vi "Send Configure Alarms.vi"(6 "Boolean Alarm Controls":T1, 7 "Message Priority (Normal)":T3=enum."Normal", 8 "error in (no error)":errorcluster, 9 "Alarm Limits":T2 {"Deadband (0.0000)" min=0.0 max=9999.9 step=0.0001 format="%.4f"; "Low Value (0.0000)" min=-9999.9 max=9999.9 step=0.0001 format="%.4f"; "High Value (0.0000)" min=-9999.9 max=9999.9 step=0.0001 format="%.4f"}, 10 "Input (0)":i32 min=0 max=7 step=1, 11 "Message Enqueuer":refnum<class "Message Enqueuer.lvclass">) -> (0 "error out":errorcluster, 3 "Message Enqueuer out":refnum<class "Message Enqueuer.lvclass">)   [LabVIEW 2016, in "LS218.lvlib" / "Configure Alarms Msg.lvclass"]
doc: "Sends the <B>LS218.lvlib:Configure Alarms Msg.lvclass</B> message.\n\n<B>LS218.lvlib:LS218.lvclass:Configure Alarms.vi</B> Description:\n\nThis VI configures all alarm functions for the selected input. Alarm functions include source, on/off, high value, low value, deadband, and latching parameters. This VI also enables/disables the system beeper, this control applies to all inputs."
uses:
  Configure Alarms Msg.lvclass
  <vilib>/ActorFramework/Message Enqueuer/Message Enqueuer.lvclass
  <vilib>/ActorFramework/Message Enqueuer/Message Priority.ctl
  C:/Program Files (x86)/National Instruments/LabVIEW 2016/vi.lib/ActorFramework/Message/Message.lvclass
  Configure Alarms Msg.lvclass/Configure Alarms Msg.ctl
  <vilib>/ActorFramework/Message Enqueuer/Message Enqueuer.lvclass/Message Enqueuer.ctl
  <vilib>/ActorFramework/Message Priority Queue/Priority Enqueue.vi
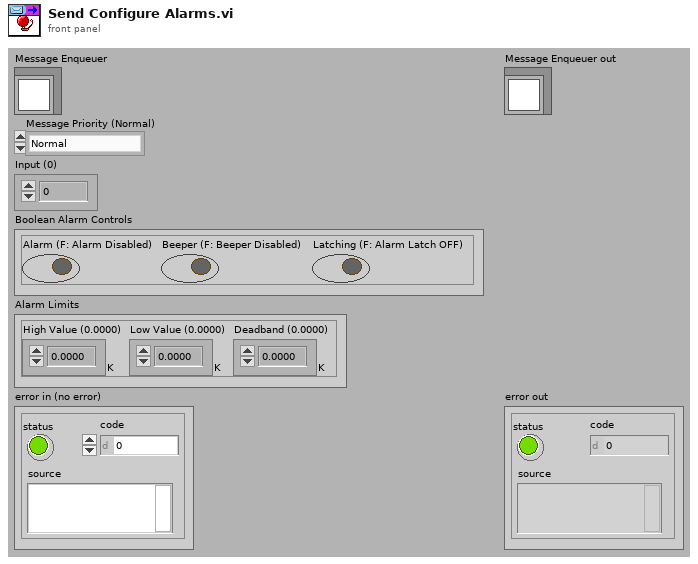
[diagram p1: front panel]
types:
  T1 = cluster{"Alarm (F: Alarm Disabled)":bool, "Beeper (F: Beeper Disabled)":bool, "Latching (F: Alarm Latch OFF)":bool}
  T2 = cluster{"High Value (0.0000)":dbl[unit], "Low Value (0.0000)":dbl[unit], "Deadband (0.0000)":dbl[unit]}
  T3 = typedef "Actor Framework.lvlib/Message Enqueuer.lvclass/Message Priority.ctl" = enum16{"Low", "Normal", "High"}
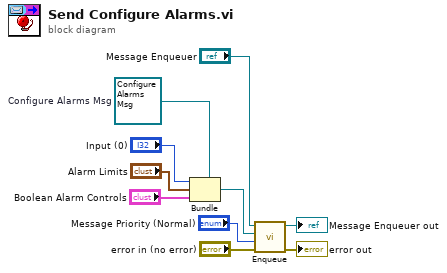
[diagram p0: block diagram]
diagram:
  w4 = refnum<class "Configure Alarms Msg.lvclass"> refnum  # Configure Alarms Msg
  n1 = Bundle(cluster=w4, "Input (0)", "Alarm Limits", "Boolean Alarm Controls") -> (w7:refnum<class "Configure Alarms Msg.lvclass">)
  n2 = call <vilib>:"Enqueue.vi"("error in (no error)"="error in (no error)", "Message Priority (Normal)"="Message Priority (Normal)", "Message"=w7, "Message Enqueuer in"="Message Enqueuer") -> ("error out"=→"error out":errorcluster, "Message Enqueuer out"=→"Message Enqueuer out":refnum<class "Message Enqueuer.lvclass">)  [unwired: 6 in]
